vi "Image buffer.vi"(4 "MASTER in":T1 {"Image data"."Color Palette" items=["Grayscale U8", "False Color", "Overexposed"]; "Image data"."Exposure time [us]" format="%#_10g"; "Queue"."Initial time [s]" format="%_19f"; "Queue"."Raw data [V]\n(all samples)" format="%0.2f"; "Queue"."Timestamp [s]" format="%_19f"}) -> (1 "MASTER out":T1 {"Image data"."Color Palette" items=["Grayscale U8", "False Color", "Overexposed"]; "Image data"."Exposure time [us]" format="%#_10g"; "Queue"."Initial time [s]" format="%_19f"; "Queue"."Raw data [V]\n(all samples)" format="%0.2f"; "Queue"."Timestamp [s]" format="%_19f"})   [LabVIEW 2020]
uses:
  MASTER.ctl
  Constants.ctl
  QBundle.ctl
  Queue.ctl
  Image data.ctl
  <vilib>/userdefined/High Color/IMAQdx.ctl
  <vilib>/vision/Image Controls.llb/IMAQ Image.ctl
  Image QBundle.ctl
  <resource>/objmgr/imaqdx.rc
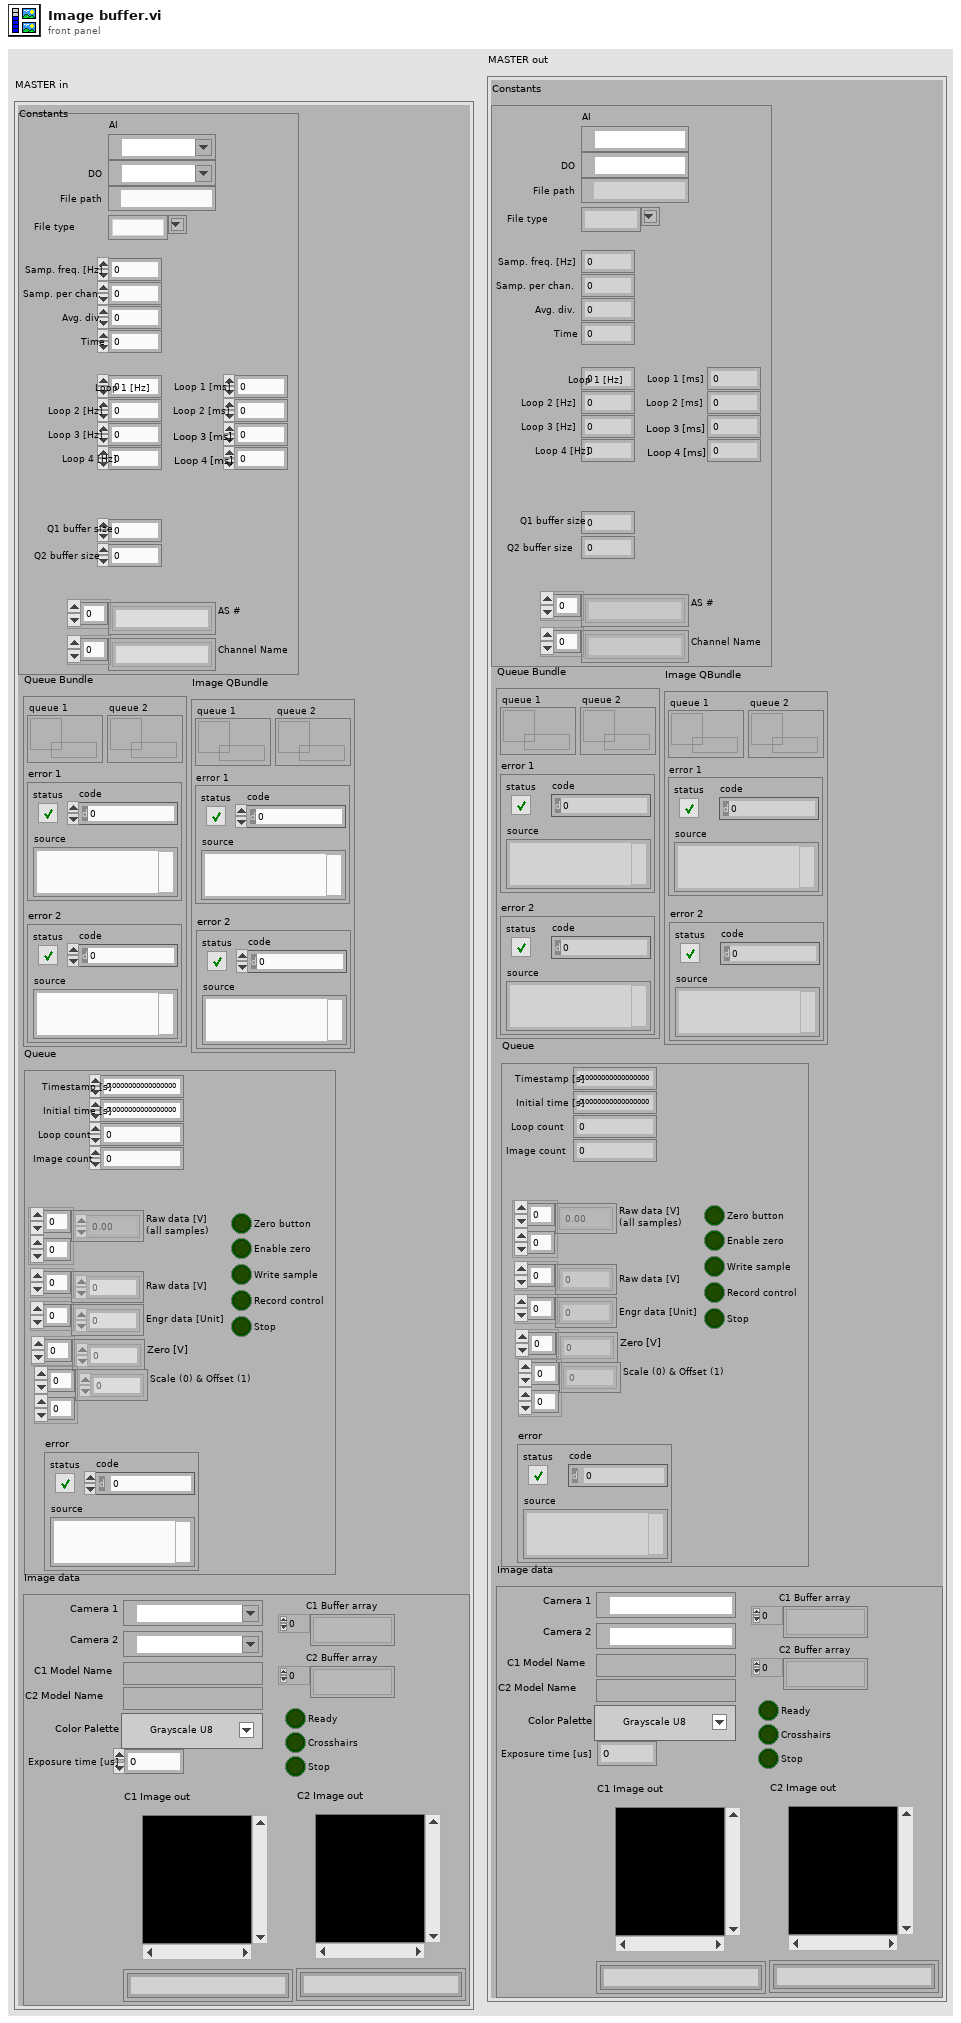
[diagram p1: front panel]
types:
  T1 = typedef "MASTER.ctl" = cluster{"Constants":T2, "Queue Bundle":T3, "Queue":T4, "Image data":T5, "Image QBundle ":T8}
  T2 = typedef "Constants.ctl" = cluster{"Time":u16, "Samp. freq. [Hz]":dbl, "Samp. per chan.":i32, "Avg. div.":i32, "File path":path, "AI":refnum<k21>, "Loop 1 [Hz]":dbl, "Loop 2 [Hz]":dbl, "Loop 3 [Hz]":dbl, "Loop 1 [ms]":dbl, "Loop 2 [ms]":dbl, "Loop 3 [ms]":dbl, "Q1 buffer size":i32, "Q2 buffer size":i32, "File type":string, "Loop 4 [Hz]":dbl, "Loop 4 [ms]":dbl, "Channel Name":string[], "AS #":string[], "DO":refnum<k21>}
  T3 = typedef "QBundle.ctl" = cluster{"queue 1":refnum<queue>, "error 1":errorcluster, "queue 2":refnum<queue>, "error 2":errorcluster}
  T4 = typedef "Queue.ctl" = cluster{"Enable zero":bool, "Engr data [Unit]":dbl[], "Zero button":bool, "Zero [V]":dbl[], "Timestamp [s]":dbl, "Write sample":bool, "Record control":bool, "Stop":bool, "error":errorcluster, "Raw data [V]\n(all samples)":dbl[][], "Raw data [V]":dbl[], "Loop count":i64, "Initial time [s]":dbl, "Scale (0) & Offset (1)":dbl[][], "Image count":dbl}
  T5 = typedef "Image data.ctl" = cluster{"Camera 1":T6, "Camera 2":T6, "C1 Image out ":T7, "C2 Image out":T7, "C1 Model Name":string, "C2 Model Name":string, "Exposure time [us]":dbl, "Color Palette":u16, "C1 Buffer array":T7[], "Ready":bool, "C2 Buffer array":T7[], "Crosshairs":bool, "Stop":bool}
  T6 = typedef "IMAQdx.ctl" = refnum<k21>
  T7 = typedef "IMAQ Image.ctl" = refnum<image>
  T8 = typedef "Image QBundle.ctl" = cluster{"queue 1":refnum<queue>, "error 1":errorcluster, "queue 2":refnum<queue>, "error 2":errorcluster}
  T9 = typedef "Image Type" = u32
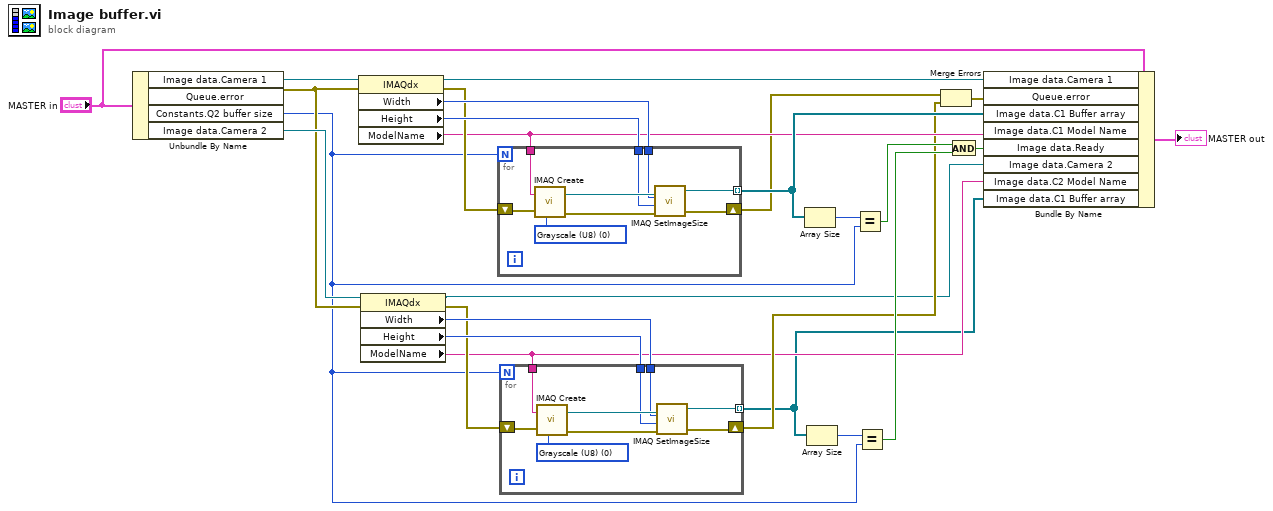
[diagram p0: block diagram]
diagram:
  n1 = Unbundle By Name("MASTER in") -> ("Image data.Camera 1"=w22:T6, "Queue.error"=w10:errorcluster, "Constants.Q2 buffer size"=w3:i32, "Image data.Camera 2"=w11:T6)
  n2 = property class="IMAQdx"(reference=w22, error in=w10) -> (reference out=w20:T6, error out=w24:errorcluster, "Width"=w26:u32, "Height"=w25:u32, "ModelName"=w17:string)
  n3 = property class="IMAQdx"(reference=w11, error in=w10) -> (reference out=w2:T6, error out=w13:errorcluster, "Width"=w15:u32, "Height"=w14:u32, "ModelName"=w4:string)
  n4 = for {
    N: w3 -> [_]
    tunnel: w26 -> [w34]
    tunnel: w25 -> [w33]
    tunnel: w17 -> [w32]
    shift-right: [w29] -> w6
    shift-left: w24 -> [w31]
    tunnel: [w27] -> w18 mode=indexing
    w28 = T9 0 items=["Grayscale (U8)", "Grayscale (I16)", "Grayscale (SGL)", "Complex (CSG)", "RGB (U32)", "HSL (U32)", "RGB (U64)", "Grayscale (U16)"] ("Image Type")
    n5 = call "IMAQ Create"("Image Name"=w32, "Image Type"=w28, "error in (no error)"=w31) -> ("New Image"=w35:T7, "error out"=w30:errorcluster)  [unwired: 1 in, 1 out]
    n6 = call "IMAQ SetImageSize"("error in (no error)"=w30, "Y Resolution"=w33, "X Resolution"=w34, "Image"=w35) -> ("error out"=w29:errorcluster, "Image Out"=w27:T7)  [unwired: 1 in]
  }
  n7 = for {
    N: w3 -> [_]
    tunnel: w15 -> [w43]
    tunnel: w14 -> [w42]
    tunnel: w4 -> [w41]
    shift-right: [w38] -> w5
    shift-left: w13 -> [w40]
    tunnel: [w36] -> w1 mode=indexing
    w37 = T9 0 items=["Grayscale (U8)", "Grayscale (I16)", "Grayscale (SGL)", "Complex (CSG)", "RGB (U32)", "HSL (U32)", "RGB (U64)", "Grayscale (U16)"] ("Image Type")
    n8 = call "IMAQ Create"("Image Name"=w41, "Image Type"=w37, "error in (no error)"=w40) -> ("New Image"=w44:T7, "error out"=w39:errorcluster)  [unwired: 1 in, 1 out]
    n9 = call "IMAQ SetImageSize"("error in (no error)"=w39, "Y Resolution"=w42, "X Resolution"=w43, "Image"=w44) -> ("error out"=w38:errorcluster, "Image Out"=w36:T7)  [unwired: 1 in]
  }
  n10 = Array Size(array=w18) -> (size(s)=w23:i32)
  n11 = Array Size(array=w1) -> (size(s)=w12:i32)
  n12 = Equal?(x=w23, y=w3) -> (x = y?=w8:bool)
  n13 = Equal?(x=w12, y=w3) -> (x = y?=w9:bool)
  n14 = Merge Errors(w6, w5) -> (w7:errorcluster)
  n15 = And(x=w8, y=w9) -> (x .and. y?=w16:bool)
  n16 = Bundle By Name(cluster="MASTER in", "Image data.Camera 1"=w20, "Queue.error"=w7, "Image data.C1 Buffer array"=w18, "Image data.C1 Model Name"=w17, "Image data.Ready"=w16, "Image data.Camera 2"=w2, "Image data.C2 Model Name"=w4, "Image data.C1 Buffer array"=w1) -> (→"MASTER out":T1)
